vi "PH_Beamline.set Status Subscriber Information.vi"(0 "i ref in":refnum<vi>, 5 "error in (no error)":errorcluster) -> (14 "i ref out":refnum<vi>, 19 "error out":errorcluster)   [LabVIEW 2014, in "PH_Beamline.lvlib"]
doc: "This VI sets relevant Information for Status Subscriber."
uses:
  PH_Beamline.lvlib
  PH_BL-Master/PH_BL-Master.Status Subscriber Information.ctl
  PH_BL-Master/PH_BL-Master.Attribute Set.ctl
  PH_Beamline.Black Box Instances.ctl
  PH_Beamline.Switch Instances.ctl
  PH_Beamline.Switch+6P Instances.ctl
  PH_Beamline.6P Switch Instances.ctl
  PH_Beamline.Switch GUI Instances.ctl
  PH_Beamline.Force Sensor Instances.ctl
  PH_BL-Master/PH_BL-Master.lvlib
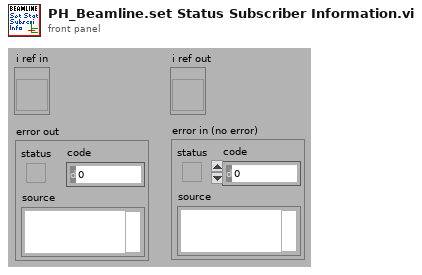
[diagram p1: front panel]
types:
  T1 = typedef "PH_Beamline.lvlib/PH_Beamline.i attribute.ctl" = cluster{"GUI Refs":cluster{"PA ok":refnum<vi>, "MA ok":refnum<vi>, "fs FE ok":refnum<vi>, "ns FE ok":refnum<vi>, "PA ED ok":refnum<vi>, "MAS ok":refnum<vi>, "Booster ok":refnum<vi>, "Mirrortower ok":refnum<vi>, "In.-Box ok":refnum<vi>, "Compressor ok":refnum<vi>, "Experiment LB ok":refnum<vi>, "Experiment LL ok":refnum<vi>, "PHELIX_Beckhoff_Watchdog":refnum<vi>, "Shutters closed":refnum<vi>, "uOPA ok":refnum<vi>, "Vacuum no shotcond Comp LB":refnum<vi>}, "Refs BL MA":refnum<vi>[], "Refs BL MA-IB":refnum<vi>[], "Refs BL fs":refnum<vi>[], "Refs BL PA ED":refnum<vi>[], "Refs BL MAS":refnum<vi>[], "Refs BL Boo":refnum<vi>[], "Refs BL ns":refnum<vi>[], "Refs BL Mirrortower":refnum<vi>[], "Refs BL Compressor":refnum<vi>[], "Refs BL Exp LB":refnum<vi>[], "Radiation Safety":cluster{"Exp Laserbay":cluster{"Ref Op Mode":refnum<vi>, "Ref Laserbay evacuated":refnum<vi>, "Tagname LB evacuated":string, "Shot Mode":T2, "Laserbay evacuated?":i32, "Tagname HV room locked":string, "HV room locked?":i32, "Ref HV room locked":refnum<vi>, "Tagname bridged?":string, "Ref Bridge":refnum<vi>, "I<1E18W/cm²":bool}, "Exp Laserlab":cluster{"Ref Op Mode":refnum<vi>, "Ref Laserlab evacuated":refnum<vi>, "Tagname LL evacuated":string, "Shot Mode":T2, "Laserlab evacuated?":i32, "Tagname bridged?":string, "Ref Bridge":refnum<vi>, "I<1E18W/cm²":bool}}, "Refs BL LL":refnum<vi>[], "PP Igni Heating GUI Refs":refnum<vi>[], "PP Igni Heating Tagnames ":string[], "Refs BL PA":cluster{"undelayed Line before Shutter":refnum<vi>[], "undelayed Line after Shutter":refnum<vi>[], "before Bypass":refnum<vi>[], "delayed Line before Shutter":refnum<vi>[], "delayed Line after Shutter":refnum<vi>[], "before Shutter Input":refnum<vi>[], "after Shutter Input":refnum<vi>[], "Bypass":refnum<vi>[], "before Shutter Exit":refnum<vi>[], "after Shutter Exit":refnum<vi>[], "to MA":refnum<vi>[], "to Lab":refnum<vi>[]}, "BL":cluster{"YLF_BL_Status":i32, "fs_BL_Status":i32, "fs_YLF_BL_Status":i32, "ns_BL_Status":i32, "PA_Input_BL_Status":i32, "PA_UnDelay_BL_Status":i32, "PA_Delay_BL_Status":i32, "PA_BL_Status":i32, "PA_Bypass_BL_Status":i32, "PA_Exit_BL_Status":i32, "PA_LL_BL_Status":i32, "LL_BL_Status":i32, "PA_MA_BL_Status":i32, "MA_Exit_BL_Status":i32, "MA_Z6_BL_Status":i32, "Z6_BL_Status":i32, "MA_LB_BL_Status":i32, "LB_TB2_BL_Status":i32, "PA_before_Bypass_BL_Status":i32, "LB_TB3_BL_Status":i32}, "State Subsystems":cluster{"PA":bool, "MA":bool, "ns FE":bool, "fs FE":bool, "PA ED":bool, "In.-Box":bool, "MAS":bool, "Booster":bool, "Mirrortower":bool, "Compressor":bool, "Experiment LB":bool, "Experiment LL":bool, "uOPA":bool}, "Status Subscriber Information":T3, "Refs BL uOPA":refnum<vi>[], "PA_Input_2_Beam_6PWpGUI not linked?":bool, "PA_Input_Delay_6PGUI not linked?":bool, "Settings":T6}
  T2 = typedef "PH_Beamline.lvlib/PH_Beamline.Operation Mode.ctl" = i32
  T3 = typedef "PH_Beamline.lvlib/PH_Beamline.Status Subscriber Information.ctl" = cluster{"fs Swich YLF":T4, "fs Exit Shutter":T4, "ns Exit Shutter":T4, "PA Input Shutter":T4, "PA PC WP":T4, "PA PC WP 2":T4, "PA Bypass In":T4, "PA Bypass Out":T4, "PA CH 1":T4, "PA delayed":T4, "PA non delayed":T4, "PA Exit Shutter":T4, "PA Switch Lab":T4, "PA Bridge CH Input MA":T4, "MA Diffusor IB":T4, "MA IB Ready":T4, "MA CH 1":T4, "MA CH 2":T4, "MA CH 3":T4, "MA CH 4":T4, "MA Shutter Align Cam":T4, "MA Position MM5":T4, "Calorimeter Switch":T4, "BL Z6 CH 9":T4, "BL Z6 Beamdump":T4, "BL Z6 Shutter":T4, "COS Sensitivity Switch":T4, "Exp LB Shutter":T4, "Exp LB TB 2":T4, "Exp LB TB 3":T4, "PA LL Input CH":T4, "PA LL Output CH":T4, "LL Comp Input Shutter":T4, "LL Comp Output Shutter":T4, "LL Comp FF Shutter":T4, "Exp LL Shutter":T4, "MA IM In IB":T4, "MA IM Out IB":T4, "MA DB In IB":T4, "MA DB Out IB":T4, "Exp LB Shutter Interlock":T4, "Exp LL Shutter Interlock":T4, "MM1 Force Sensor":T4}
  T4 = typedef "PH_BL-Master.lvlib/PH_BL-Master.Status Subscriber Information.ctl" = cluster{"Index of element":i32, "Attributeset":T5}
  T5 = typedef "PH_BL-Master.lvlib/PH_BL-Master.Attribute Set.ctl" = enum16{"Boolean Status Service Subscriber", "Picture Status Service Subscriber"}
  T6 = typedef "PH_Beamline_Chief.lvlib/PH_Beamline_Chief.Settings.ctl" = cluster{"PA Doublepass Mode":bool, "Compressor Vaccuum LB not relevant":bool, "Windowshutter TB2 not relevant":bool, "Windowshutter TB3 not relevant":bool}
  T7 = typedef "PH_Beamline.lvlib/PH_Beamline.Force Sensor Instances.ctl" = string
  T8 = typedef "PH_Beamline.lvlib/PH_Beamline.Switch GUI Instances.ctl" = string
  T9 = typedef "PH_Beamline.lvlib/PH_Beamline.Switch Instances.ctl" = string
  T10 = typedef "PH_Beamline.lvlib/PH_Beamline.Black Box Instances.ctl" = string
  T11 = typedef "PH_Beamline.lvlib/PH_Beamline.6P Switch Instances.ctl" = string
  T12 = typedef "PH_Beamline.lvlib/PH_Beamline.Switch+6P Instances.ctl" = string
  T13 = cluster{"[0]":T4, "[1]":T4, "[2]":T4, "[3]":T4, "[4]":T4, "[5]":T4, "[6]":T4, "[7]":T4, "[8]":T4, "[9]":T4, "[10]":T4, "[11]":T4, "[12]":T4, "[13]":T4, "[14]":T4, "[15]":T4, "[16]":T4, "[17]":T4, "[18]":T4, "[19]":T4, "[20]":T4, "[21]":T4, "[22]":T4, "[23]":T4, "[24]":T4, "[25]":T4, "[26]":T4, "[27]":T4, "[28]":T4, "[29]":T4, "[30]":T4, "[31]":T4, "[32]":T4, "[33]":T4, "[34]":T4, "[35]":T4, "[36]":T4, "[37]":T4, "[38]":T4, "[39]":T4, "[40]":T4, "[41]":T4, "[42]":T4}
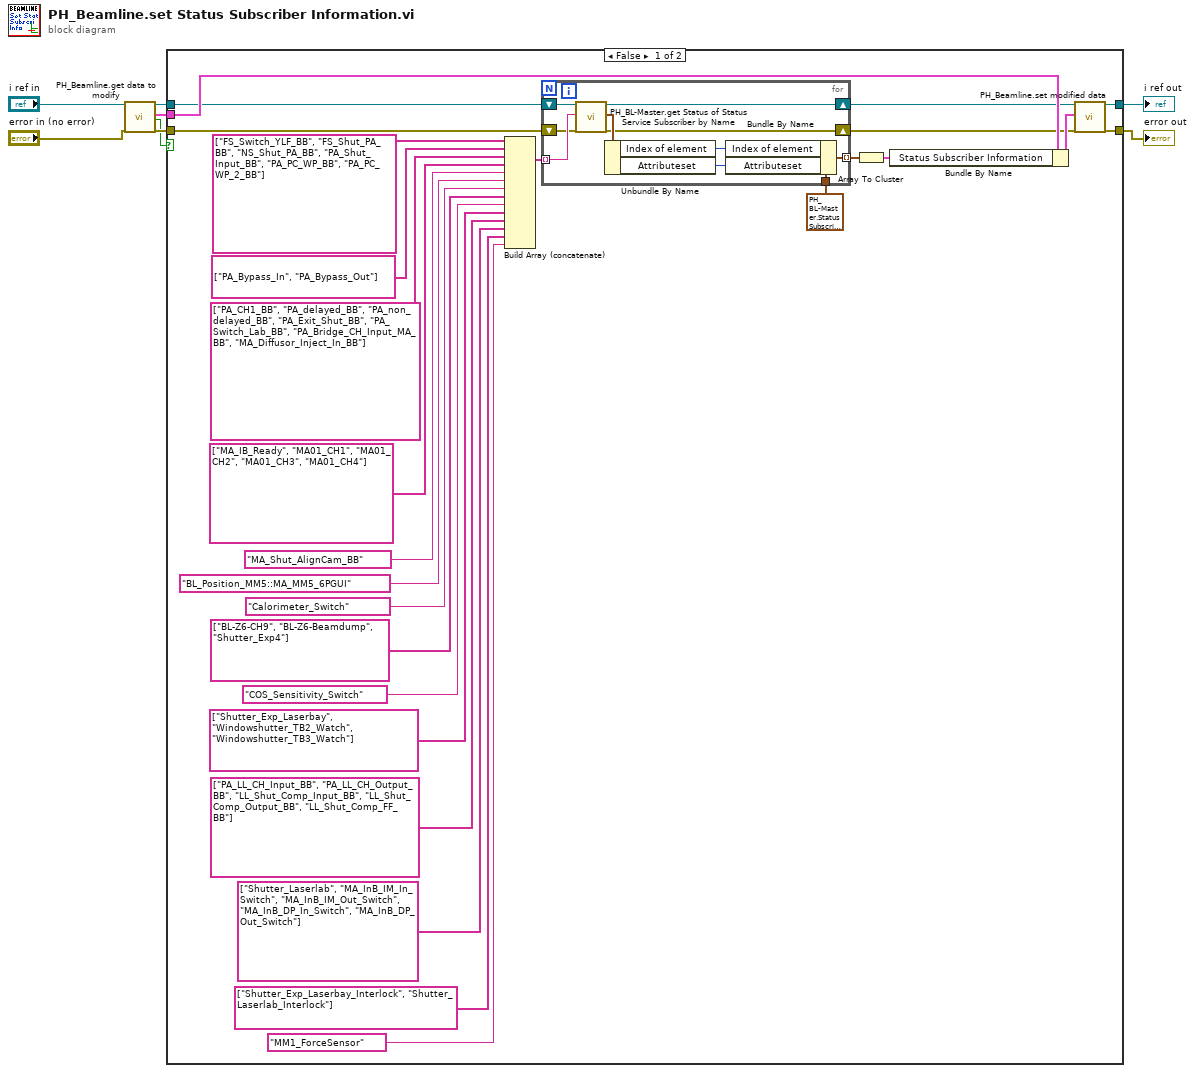
[diagram p0: block diagram]
diagram:
  n1 = call "PH_Beamline.get data to modify.vi"("i ref in"="i ref in", "error in (no error)"="error in (no error)") -> ("i ref out"=w6:refnum<vi>, "i attribute"=w2:T1, "timed out"=w3:bool, "error out"=w4:errorcluster)  [unwired: 14 in]
  n2 = case shown="False" w3 {
    tunnel: w6 -> [w15 w46]
    tunnel: [w34 w46] -> w5
    tunnel: w4 -> [w13 w45]
    tunnel: w2 -> [w16 _]
    tunnel: [w32 w45] -> w1
    frame False {
      n3 = Build Array (concatenate)(T10[] ["FS_Switch_YLF_BB", "FS_Shut_PA_BB", "NS_Shut_PA_BB", "PA_Shut_Input_BB", "PA_PC_WP_BB", "PA_PC_WP_2_BB"], T9[] ["PA_Bypass_In", "PA_Bypass_Out"], T10[] ["PA_CH1_BB", "PA_delayed_BB", "PA_non_delayed_BB", "PA_Exit_Shut_BB", "PA_Switch_Lab_BB", "PA_Bridge_CH_Input_MA_BB", "MA_Diffusor_Inject_In_BB"], T9[] ["MA_IB_Ready", "MA01_CH1", "MA01_CH2", "MA01_CH3", "MA01_CH4"], T10 "MA_Shut_AlignCam_BB" ("Black Box Instances"), T12 "BL_Position_MM5::MA_MM5_6PGUI" ("Switch and 6P Instances"), T11 "Calorimeter_Switch" ("6P Switch Instances"), T9[] ["BL-Z6-CH9", "BL-Z6-Beamdump", "Shutter_Exp4"], T11 "COS_Sensitivity_Switch" ("6P Switch Instances"), T9[] ["Shutter_Exp_Laserbay", "Windowshutter_TB2_Watch", "Windowshutter_TB3_Watch"], T10[] ["PA_LL_CH_Input_BB", "PA_LL_CH_Output_BB", "LL_Shut_Comp_Input_BB", "LL_Shut_Comp_Output_BB", "LL_Shut_Comp_FF_BB"], T9[] ["Shutter_Laserlab", "MA_InB_IM_In_Switch", "MA_InB_IM_Out_Switch", "MA_InB_DP_In_Switch", "MA_InB_DP_Out_Switch"], T8[] ["Shutter_Exp_Laserbay_Interlock", "Shutter_Laserlab_Interlock"], T7 "MM1_ForceSensor" ("Force Sensor Instances")) -> (w28:T7[])
      n4 = for {
        tunnel: T4 {"Index of element"=0, "Attributeset"=enum."Boolean Status Service Subscriber"} ("Status Subscriber Information.fs Exit Shutter") -> [w44]
        tunnel: [w43] -> w31 mode=indexing
        tunnel: w28 -> [w39] mode=indexing
        shift-right: [w36] -> w14
        shift-left: w15 -> [w38]
        shift-right: [w35] -> w12
        shift-left: w13 -> [w37]
        n5 = call "PH_BL-Master.get Status of Status Service Subscriber by Name.vi"("i ref in"=w38, "Status Subscriber Instance"=w39, "error in (no error)"=w37) -> ("i ref out"=w36:refnum<vi>, "Status Subscriber Information"=w42:T4, "error out"=w35:errorcluster)  [unwired: 14 in]
        n6 = Unbundle By Name(w42) -> ("Index of element"=w41:i32, "Attributeset"=w40:T5)
        n7 = Bundle By Name(cluster=w44, "Index of element"=w41, "Attributeset"=w40) -> (w43:T4)
      }
      n8 = Array To Cluster(array=w31) -> (cluster=w29:T13)
      n9 = Bundle By Name(cluster=w16, "Status Subscriber Information"=w29) -> (w33:T1)
      n10 = call "PH_Beamline.set modified data.vi"("i ref in"=w14, "i attribute"=w33, "error in (no error)"=w12) -> ("i ref out"=w34:refnum<vi>, "error out"=w32:errorcluster)  [unwired: 15 in]
    }
    frame True {
    }
  }
  "i ref out" <- w5
  "error out" <- w1
